vi "Filter_Lowpass.vi"(1 "Filter":bool=TRUE, 2 "Pulse signal in":dbl[](array[numeric]), 3 "low cutoff freq: fl":dbl=40.0 format="%0.2f") -> (7 "Signal out":dbl[](array[numeric]))   [LabVIEW 2023]
uses:
  <vilib>/Analysis/3filter.llb/Filter Passband Type.ctl
  <vilib>/Analysis/4window.llb/windowTd.ctl
  <vilib>/Analysis/3filter.llb/FIR Windowed Filter (DBL).vi
  <vilib>/Analysis/NI_AALBase.lvlib
  <vilib>/Analysis/NI_AALPro.lvlib
panel:
  out "Pulse signal graph in":dbl[](graph)
  out "Pulse signal graph out":dbl[](graph)
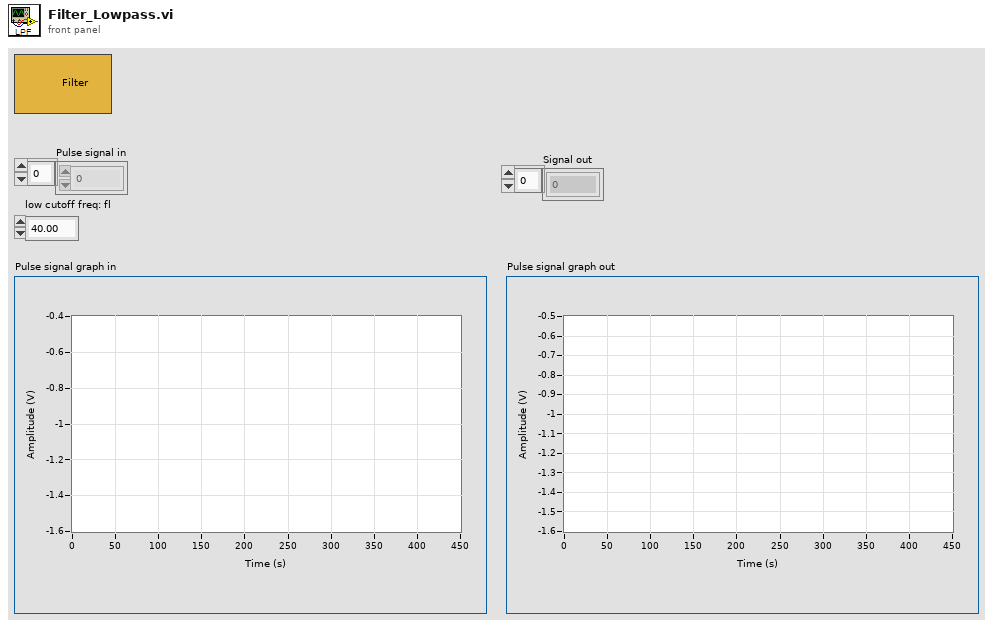
[diagram p1: front panel]
types:
  T1 = typedef "NI_AALBase.lvlib/Filter Passband Type.ctl" = enum32{"Lowpass", "Highpass", "Bandpass", "Bandstop"}
  T2 = typedef "NI_AALPro.lvlib/windowTd.ctl" = u32
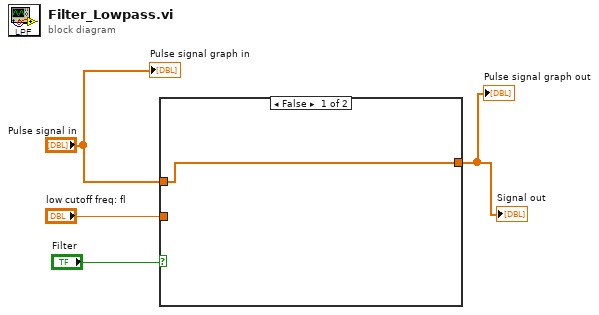
[diagram p0: block diagram]
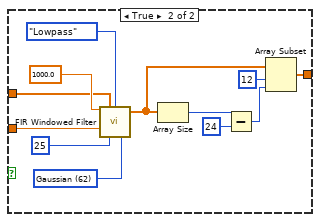
[diagram p2: hidden frame]
diagram:
  n1 = case shown="False" "Filter" {
    tunnel: "low cutoff freq: fl" -> [_ w10]
    tunnel: "Pulse signal in" -> [w5 w8]
    tunnel: [w5 w6] -> w2
    frame False {
    }
    frame True {
      w11 = T2 62 items=["Rectangle"=0, "Hanning"=1, "Hamming"=2, "Blackman-Harris"=3, "Exact Blackman"=4, "Blackman"=5, "Flat Top"=6, "4 Term B-Harris "=7, "7 Term B-Harris"=8, "Low Sidelobe"=9, "Blackman Nuttall"=11, "Triangle"=30, "Bartlett-Hanning"=31, "Bohman"=32, "Parzen"=33, "Welch"=34, "Kaiser"=60, "Dolph-Chebyshev"=61, "Gaussian"=62] ("window")
      n2 = call-poly <vilib>:"FIR Windowed Filter.vi"("sampling freq: fs"=1000.0, "X"=w8, "filter type"=Filter_Passband_Type."Lowpass", "low cutoff freq: fl"=w10, "taps"=25, "window"=w11) -> ("Filtered X"=w7:dbl[])  [unwired: 8 in, 1 out]
      n3 = Array Size(array=w7) -> (size(s)=w9:i32)
      n4 = Subtract(x=w9, y=24) -> (x-y=w13:i32)
      n5 = Array Subset(array=w7, index=12, length=w13) -> (w6:dbl[])
    }
  }
  "Pulse signal graph out" <- w2
  "Signal out" <- w2
  "Pulse signal graph in" <- "Pulse signal in"
